vi "MoveVelocity.vi"(0 "Side":T1=enum."right", 1 "node":string, 2 "Arm Velocities":T2, 3 "error in":errorcluster) -> (6 "error out":errorcluster)   [LabVIEW 2010]
uses:
  ROS/Code/SubVIs/JointMode.ctl
  ROS/Code/SubVIs/BaxterArmsSmall.ctl
  ROS/Code/SubVIs/BaxterSide.ctl
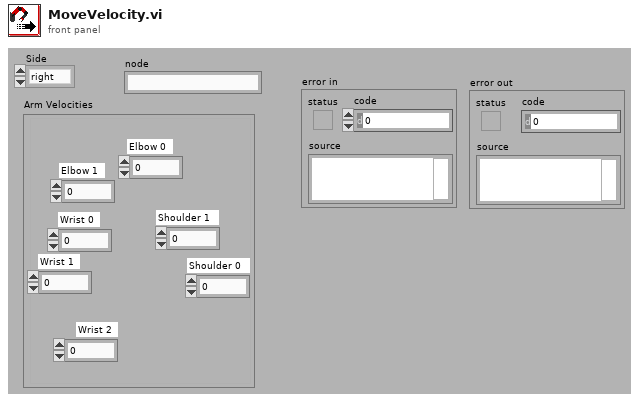
[diagram p1: front panel]
types:
  T1 = typedef "BaxterSide.ctl" = enum16{"left", "right"}
  T2 = typedef "BaxterArmsSmall.ctl" = cluster{"Elbow 0":dbl, "Elbow 1":dbl, "Shoulder 0":dbl, "Shoulder 1":dbl, "Wrist 0":dbl, "Wrist 1":dbl, "Wrist 2":dbl}
  T3 = typedef "JointMode.ctl" = u8
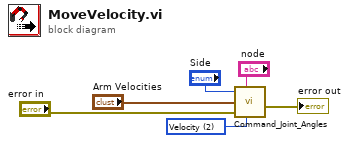
[diagram p0: block diagram]
diagram:
  w6 = T3 2 items=["Position"=1, "Velocity"=2, "Effort"=3] ("Mode")
  n1 = call "Command_Joint_Angles.vi"("Side"="Side", "node"="node", "Arm Angles (degrees)"="Arm Velocities", "error in"="error in", "Mode"=w6) -> ("error out"=→"error out":errorcluster)  [unwired: 1 in]
